vi "Lab_2_Calculate_HR_Zones.vi"(8 "Error IN":errorcluster, 11 "HR Data Structure IN":T1 {"Raw Data"."Time" format="%<%x %.3X>T"}) -> (0 "Error OUT":errorcluster, 3 "HR Data Structure OUT":T1 {"Raw Data"."Time" format="%<%x %.3X>T"})   [LabVIEW 2025]
uses:
  HR_Data_Structure.ctl
  Raw_Data_IN_HR.ctl
  Runner_Data_Structure.ctl
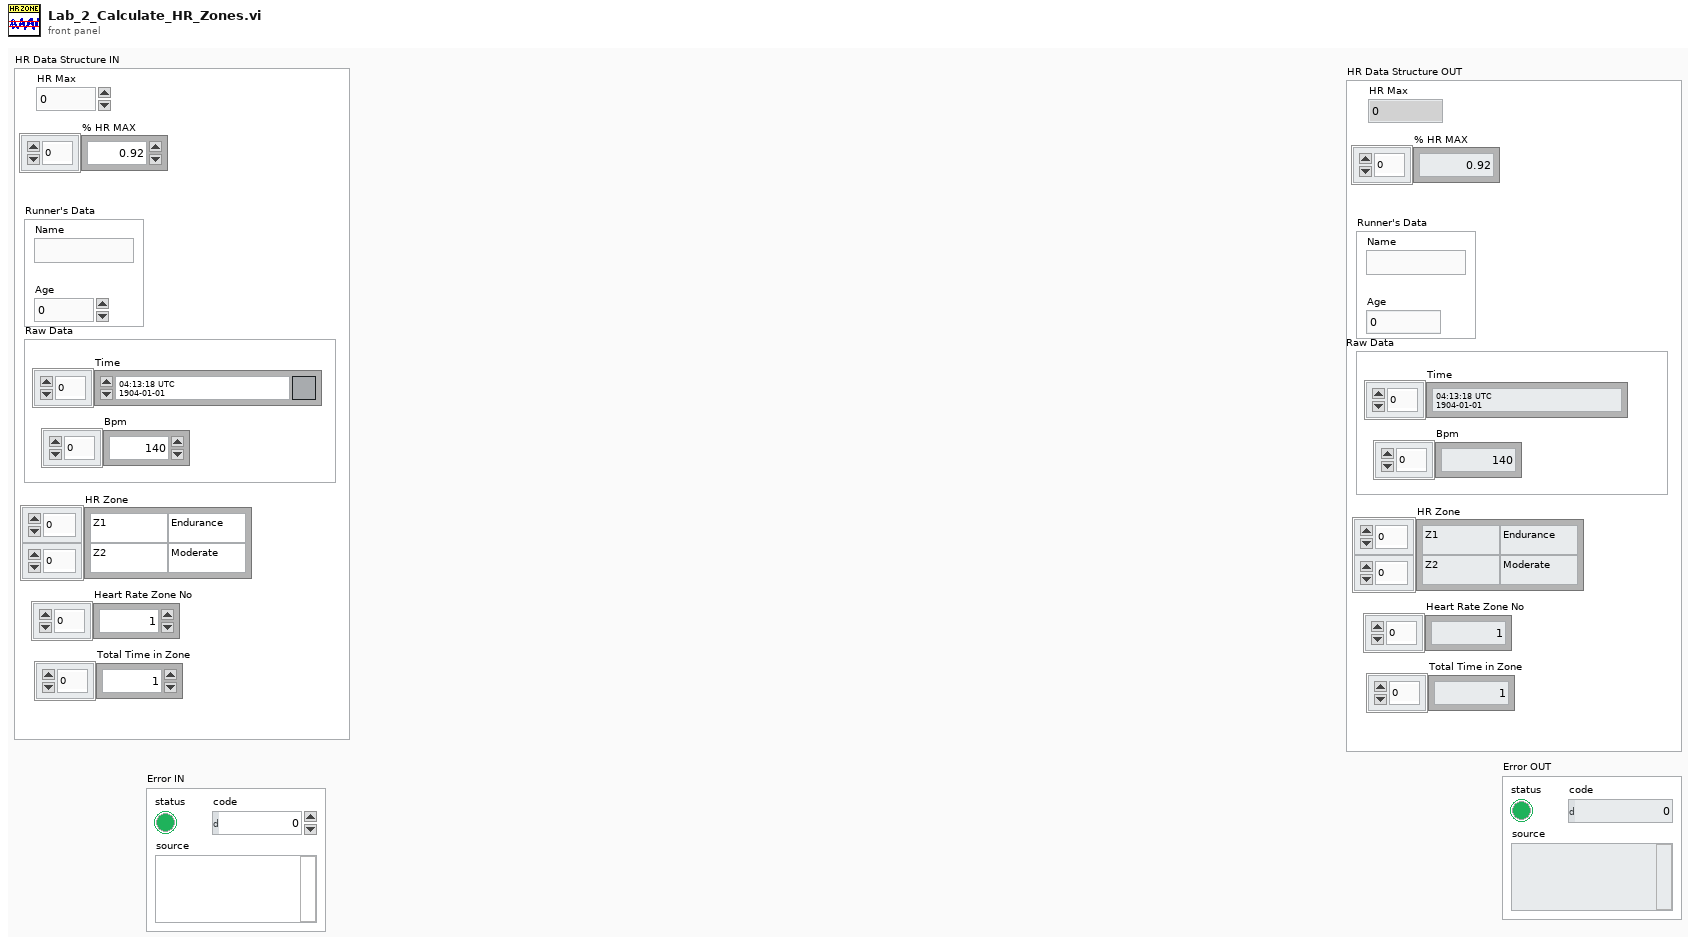
[diagram p1: front panel]
types:
  T1 = typedef "HR_Data_Structure.ctl" = cluster{"HR Max":i32, "% HR MAX ":dbl[], "Raw Data":T2, "Runner's Data":T3, "HR Zone":string[][], "Total Time in Zone":dbl[], "Heart Rate Zone No":dbl[]}
  T2 = typedef "Raw_Data_IN_HR.ctl" = cluster{"Time":timestamp[], "Bpm":i32[]}
  T3 = typedef "Runner_Data_Structure.ctl" = cluster{"Name":string, "Age":i32}
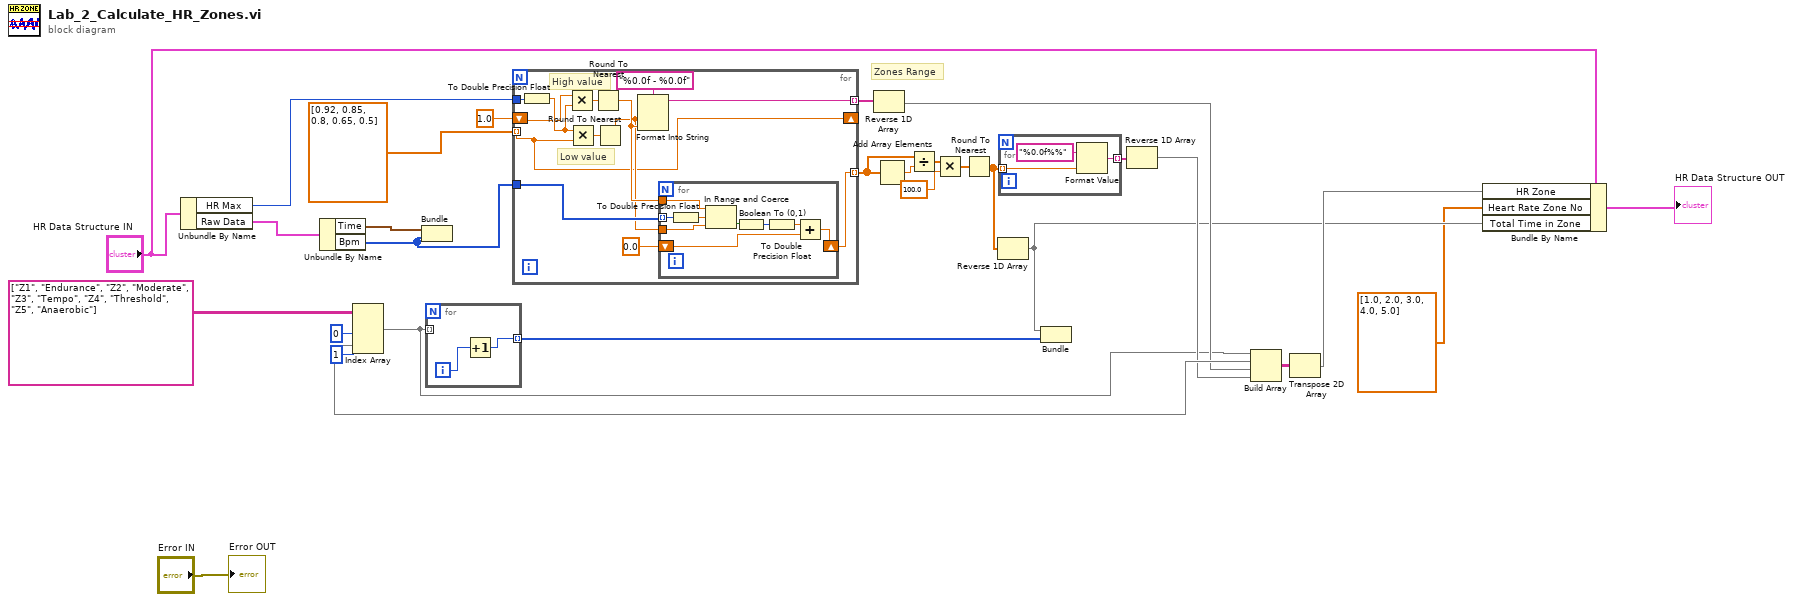
[diagram p0: block diagram]
diagram:
  # "Zones Range"
  n1 = Unbundle By Name("HR Data Structure IN") -> ("HR Max"=w4:i32, "Raw Data"=w6:T2)
  n2 = Unbundle By Name(w6) -> ("Time"=w12:timestamp[], "Bpm"=w11:i32[])
  n3 = Index Array(array=string[][] [["Z1", "Endurance"], ["Z2", "Moderate"], ["Z3", "Tempo"], ["Z4", "Threshold"], ["Z5", "Anaerobic"]], index (col) #1=0 ("index (col)"), index (col) #2=1 ("index (col)")) -> (element #1=w18:string[], element #2=w22:string[])  [unwired: 2 in]
  n4 = Bundle("Time"=w12, "Bpm"=w11) -> ()  [unwired: 1 in, 1 out]
  n5 = for {
    tunnel: w18 -> [_] mode=indexing
    tunnel: [w30] -> w17 mode=indexing
    i -> [w31]
    n6 = Increment(x=w31) -> (x+1=w30:i32)
  }
  n7 = for {
    tunnel: w4 -> [w44]
    tunnel: dbl[] [0.92, 0.85, 0.8, 0.65, 0.5] -> [w32] mode=indexing
    tunnel: [w39] -> w29 mode=indexing
    tunnel: w11 -> [w38]
    tunnel: [w34] -> w15 mode=indexing
    shift-right: [w32] -> _
    shift-left: 1.0 -> [w33]
    # "Low value"
    # "High value"
    n8 = To Double Precision Float(number=w44) -> (double precision float=w43:dbl)
    n9 = Multiply(x=w33, y=w43) -> (x*y=w42:dbl)
    n10 = Multiply(x=w43, y=w32) -> (x*y=w41:dbl)
    n11 = Round To Nearest(number=w42) -> (nearest integer value=w37:dbl)
    n12 = Round To Nearest(number=w41) -> (nearest integer value=w36:dbl)
    n13 = Format Into String(format string="%0.0f - %0.0f", w36, w37) -> (resulting string=w39:string)  [unwired: 2 in, 1 out]
    n14 = for {
      tunnel: w38 -> [w51] mode=indexing
      tunnel: w37 -> [w53]
      tunnel: w36 -> [w52]
      shift-right: [w48] -> w34
      shift-left: 0.0 -> [w49]
      n15 = To Double Precision Float(number=w51) -> (double precision float=w50:dbl)
      n16 = In Range and Coerce(upper limit=w53, x=w50, lower limit=w52) -> (In Range?=w47:bool)  [unwired: 1 out]
      n17 = Boolean To (0,1)(Boolean=w47) -> (0, 1=w46:i16)
      n18 = To Double Precision Float(number=w46) -> (double precision float=w45:dbl)
      n19 = Add(x=w45, y=w49) -> (x+y=w48:dbl)
    }
  }
  n20 = Reverse 1D Array(array=w29) -> (reversed array=w21:string[])
  n21 = Add Array Elements(numeric array=w15) -> (sum=w14:dbl)
  n22 = Divide(x=w15, y=w14) -> (x/y=w26:dbl[])
  n23 = Multiply(x=w26, y=100.0) -> (x*y=w25:dbl[])
  n24 = Round To Nearest(number=w25) -> (nearest integer value=w16:dbl[])
  n25 = Reverse 1D Array(array=w16) -> (reversed array=w7:dbl[])
  n26 = for {
    tunnel: w16 -> [w56] mode=indexing
    tunnel: [w54] -> w27 mode=indexing
    n27 = Format Value(format string="%0.0f%%", value (0)=w56) -> (output string=w54:string)  [unwired: 1 in]
  }
  n28 = Bundle(w7, w17) -> ()  [unwired: 1 in, 1 out]
  n29 = Reverse 1D Array(array=w27) -> (reversed array=w19:string[])
  n30 = Build Array(w18, w22, w21, w19) -> (w20:string[][])
  n31 = Transpose 2D Array(2D array=w20) -> (transposed array=w8:string[][])
  n32 = Bundle By Name(cluster="HR Data Structure IN", "HR Zone"=w8, "Heart Rate Zone No"=dbl[] [1.0, 2.0, 3.0, 4.0, 5.0], "Total Time in Zone"=w7) -> (→"HR Data Structure OUT":T1)
  "Error OUT" <- "Error IN"
